vi "Configure Multi Eval Meas Limit SEM EN-DC.vi"(0 "VISA resource name":refnum<visa-resource-name>, 1 "Frequency Start (0Hz)":dbl format="%#.9p", 2 "Level (0.0)":dbl format="%^.3e", 5 "Instance (1)":T2=1, 7 "Area (1)":T1=1, 9 "Enable (Off)":bool, 11 "error in (no error)":errorcluster, 12 "Frequency End (0Hz)":dbl format="%#.9p", 13 "RBW (30 kHz)":i32(ring) items=["30 kHz", "100 kHz", "1 MHz", "1 % of channel bandwidth", "2 % of channel bandwidth"]) -> (4 "VISA resource name out":refnum<visa-resource-name>, 15 "error out":errorcluster)   [LabVIEW 2020, in "Rohde&Schwarz CMWXP NR FR1 Measurement.lvlib"]
doc: "Defines general requirements for the emission mask area number <no> (for EN-DC). The activation state, the area borders, an upper limit and the resolution bandwidth must be specified.\n\nAttribute:\nRSCMWXPNRFR1M_ATTR_MULTI_EVAL_MEAS_LIMIT_SEM_EN_DC\n\nRemote-control command:\nCONFigure:NRSub:MEAS<i>:MEValuation:LIMit:SEMask:AREA<no>:ENDC"
uses:
  <instrlib>/Rohde&Schwarz CMWXP NR FR1 Measurement/Rohde&Schwarz CMWXP NR FR1 Measurement.lvlib
  <instrlib>/Rohde&Schwarz CMWXP NR FR1 Measurement/Private/_Instance.ctl
  <instrlib>/Rohde&Schwarz CMWXP NR FR1 Measurement/Private/_Area.ctl
  <instrlib>/Rohde&Schwarz CMWXP NR FR1 Measurement/Private/rsidr_core.llb/rsidr_core.lvlib
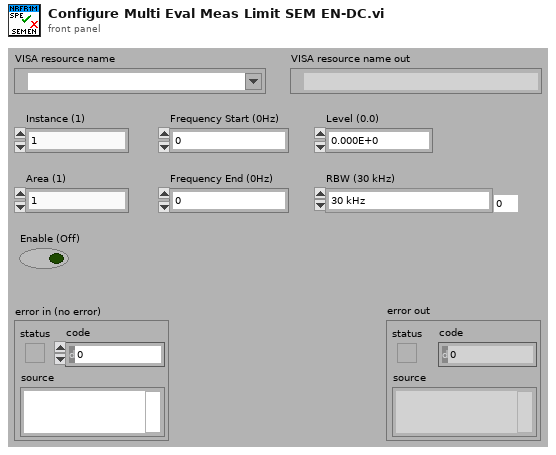
[diagram p1: front panel]
types:
  T1 = typedef "Rohde&Schwarz CMWXP NR FR1 Measurement.lvlib/_Area.ctl" = i32
  T2 = typedef "Rohde&Schwarz CMWXP NR FR1 Measurement.lvlib/_Instance.ctl" = i32
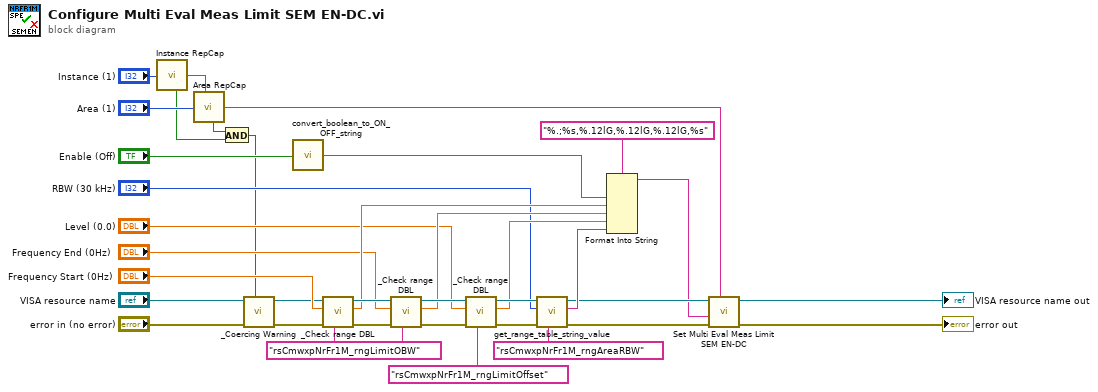
[diagram p0: block diagram]
diagram:
  w15 = "rsCmwxpNrFr1M_rngLimitOBW" ("Range Table Identifier")
  n1 = call <instrlib>:"Instance RepCap.vi"("Instance In"="Instance (1)") -> ("In Range?"=w6:bool, "RepCap Identifier Out"=w32:string)  [unwired: 1 in]
  n2 = call <instrlib>:"Area RepCap.vi"("SEM Area In"="Area (1)", "RepCap String In (\"\")"=w32) -> ("In Range?"=w7:bool, "RepCap Identifier Out"=w31:string)
  n3 = And(x=w7, y=w6) -> (x .and. y?=w1:bool)
  n4 = call <instrlib>:"_Coercing Warning.vi"("In Range?"=w1, "error in (no error)"="error in (no error)", "VISA resource name"="VISA resource name") -> ("error out"=w3:errorcluster, "VISA resource name out"=w2:refnum<visa-resource-name>)  [unwired: 7 in]
  n5 = call <instrlib>:"convert_boolean_to_ON_OFF_string.vi"("boolean value in"="Enable (Off)") -> ("string value out"=w28:string)  [unwired: 4 in]
  n6 = call <instrlib>:"_Check range DBL.vi"("Range Table Identifier"=w15, "error in (no error)"=w3, "DBL Value In"="Frequency Start (0Hz)", "VISA resource name"=w2) -> ("error out"=w27:errorcluster, "DBL Value Out"=w20:dbl, "VISA resource name out"=w26:refnum<visa-resource-name>)  [unwired: 5 in]
  n7 = call <instrlib>:"_Check range DBL.vi"("Range Table Identifier"=w15, "error in (no error)"=w27, "DBL Value In"="Frequency End (0Hz)", "VISA resource name"=w26) -> ("error out"=w25:errorcluster, "DBL Value Out"=w18:dbl, "VISA resource name out"=w24:refnum<visa-resource-name>)  [unwired: 5 in]
  n8 = call <instrlib>:"_Check range DBL.vi"("Range Table Identifier"="rsCmwxpNrFr1M_rngLimitOffset", "error in (no error)"=w25, "DBL Value In"="Level (0.0)", "VISA resource name"=w24) -> ("error out"=w23:errorcluster, "DBL Value Out"=w16:dbl, "VISA resource name out"=w22:refnum<visa-resource-name>)  [unwired: 5 in]
  n9 = call <instrlib>:"get_range_table_string_value.vi"("Range Table ID in"="rsCmwxpNrFr1M_rngAreaRBW", "error in"=w23, "I32 input"="RBW (30 kHz)", "VISA resource name"=w22) -> ("error out"=w9:errorcluster, "String Value out"=w11:string, "VISA resource name out"=w10:refnum<visa-resource-name>)  [unwired: 5 in]
  n10 = Format Into String(format string="%.;%s,%.12lG,%.12lG,%.12lG,%s", w28, w20, w18, w16, w11) -> (resulting string=w8:string)  [unwired: 2 in, 1 out]
  n11 = call "Set Multi Eval Meas Limit SEM EN-DC"("Repeated Capabilities"=w31, "error in (no error)"=w9, "Multi Eval Meas Limit SEM EN-DC ()"=w8, "instrument handle"=w10) -> ("error out"=→"error out":errorcluster, "instrument handle out"=→"VISA resource name out":refnum<visa-resource-name>)  [unwired: 6 in]
